vi "2L19_IC_de_NC_m_Sdem.vi"(8 "S dem":dbl, 9 "m":dbl, 10 "Niveau de confiance":u16(ring) items=["Risque alpha bilattéral", "Risque alpha à droite", "Risque alpha à gauche"], 11 "NC":dbl format="%.2f") -> (2 "Ic max":dbl, 3 "Ic min":dbl)   [LabVIEW 2010, in "lv_02.lvlib"]
doc: "Ce VI Calcule l'intervalle de confiance selon un Niveau de confiance NC dont le risque \n- est bilattéral (IC min, IC max) \n- est plaçé selon un risque"
uses:
  lv_02.lvlib
  1A-z-invdist.vi
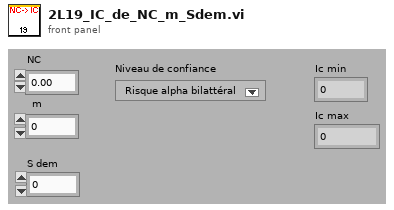
[diagram p1: front panel]
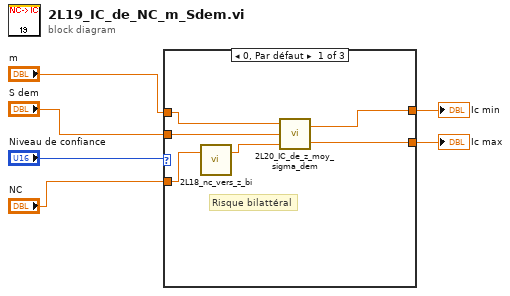
[diagram p0: block diagram]
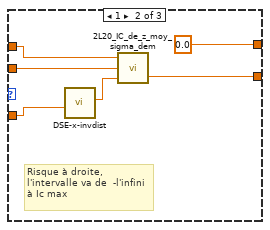
[diagram p2: hidden frame]
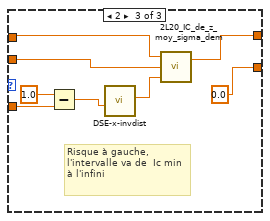
[diagram p3: hidden frame]
diagram:
  n1 = case shown="0, Par défaut" "Niveau de confiance" {
    tunnel: "NC" -> [w12 w14 w25]
    tunnel: "S dem" -> [w10 w17 w24]
    tunnel: "m" -> [w9 w18 w23]
    tunnel: [w7 w16 0.0 ("Ic max")] -> w2
    tunnel: [w8 0.0 ("Ic max") w22] -> w1
    frame 0, Default {
      # "Risque bilattéral"
      n2 = call "2L18_nc_vers_z_bi.vi"("Niveau de confiance (1- alpha)"=w12) -> ("z (apha/2)"=w11:dbl)  [unwired: 1 in, 1 out]
      n3 = call "2L20_IC_de_z_moy_sigma_dem.vi"("z"=w11, "S dem"=w10, "m"=w9) -> ("Ic max"=w7:dbl, "Ic min"=w8:dbl)
    }
    frame 1 {
      # "Risque à droite, l'intervalle va de  -l'infini à Ic max"
      n4 = call-poly "DSE-x-invdist.vi"("F(z)"=w14) -> ("z"=w13:dbl)  [unwired: 8 in, 2 out]
      n5 = call "2L20_IC_de_z_moy_sigma_dem.vi"("z"=w13, "S dem"=w17, "m"=w18) -> ("Ic max"=w16:dbl)  [unwired: 1 out]
    }
    frame 2 {
      # "Risque à gauche, l'intervalle va de  Ic min à l'infini"
      n6 = Subtract(x=1.0, y=w25) -> (x-y=w20:dbl)
      n7 = call-poly "DSE-x-invdist.vi"("F(z)"=w20) -> ("z"=w19:dbl)  [unwired: 8 in, 2 out]
      n8 = call "2L20_IC_de_z_moy_sigma_dem.vi"("z"=w19, "S dem"=w24, "m"=w23) -> ("Ic min"=w22:dbl)  [unwired: 1 out]
    }
  }
  "Ic max" <- w2
  "Ic min" <- w1
